vi "PicoScope6000aGetStreamingValues.vi"(0 "handle in":i16=16384, 1 "Polling time ms":u32=10, 2 "Buffer and Transfer Settings":T5={"startIndex"=0, "Samples"=1000000, "Down Sample Ratio"=1, "Down-Sample Mode"=2147483648} {"Down-Sample Mode" items=["RAW none"=2147483648, "None"=0, "Aggregate"=1, "Decimate"=2, "Average"=4]; "Down Sample Ratio" step=1; "Samples" format="%_6p"}, 3 "enabled array":i16[](array[numeric])=[1, 1, 0, 0, 0, 0, 0, 0, 0, 0], 5 "Device Info":T2, 7 "Data Pointers In":T3, 9 "No of Buffers":i32=1, 11 "error in (no error)":errorcluster, 13 "LoopFlag":bool) -> (4 "handle out":i16=16384, 8 "Data Pointers Out":T3, 14 "tPicoStreamingDataTriggerInfo":T1(array[cluster]), 15 "error out":errorcluster)   [LabVIEW 2010]
doc: "Call ps6000aGetValues to fill all buffers"
uses:
  ps6000a.dll
  shared/PicoBuffers.ctl
  shared/Buffer and Transfer Settings.ctl
panel:
  out "handle RunStreaming":i16
  out "error out RunStreaming":errorcluster
  out "No of channels":u64=2
  in  "tPicoStreamingDataInfo":T4={"Channel"=0, "Down-Sample Mode"=2147483648, "PICO_DATA_TYPE"=enum."PICO_INT16_T", "Samples"=0, "bufferIndex"=0, "startIndex"=0, "overflow"=0} {"overflow" step=1 format="%010b"; "Down-Sample Mode" items=["None"=2147483648, "Aggregate"=1, "Decimate"=2, "Average"=4]; "Channel" items=["Channel A"=0, "Channel B"=1, "Channel C"=2, "Channel D"=3, "Channel E"=4, "Channel F"=5, "Channel G"=6, "Channel H"=7, "Port 0"=128, "Port 1"=129, "Trigger AUX"=1001]; "startIndex" step=1}
  in  "SetDataBuffer0 flag":bool
  in  "Streaming Acquisition Settings":T6={"preTriggerSamples"=0, "postTriggerSamples"=1000000, "Requested sampleInterval"=1.0, "sampleIntervalTimeUnits"=3} {"sampleIntervalTimeUnits" items=["femtoseconds", "picoseconds", "nanoseconds", "microseconds", "millseconds", "seconds"]; "postTriggerSamples" format="%_6p"; "preTriggerSamples" format="%_6p"}
  # "Samples can be equal to or less\nTotal Pre and Post Trigger Samples"
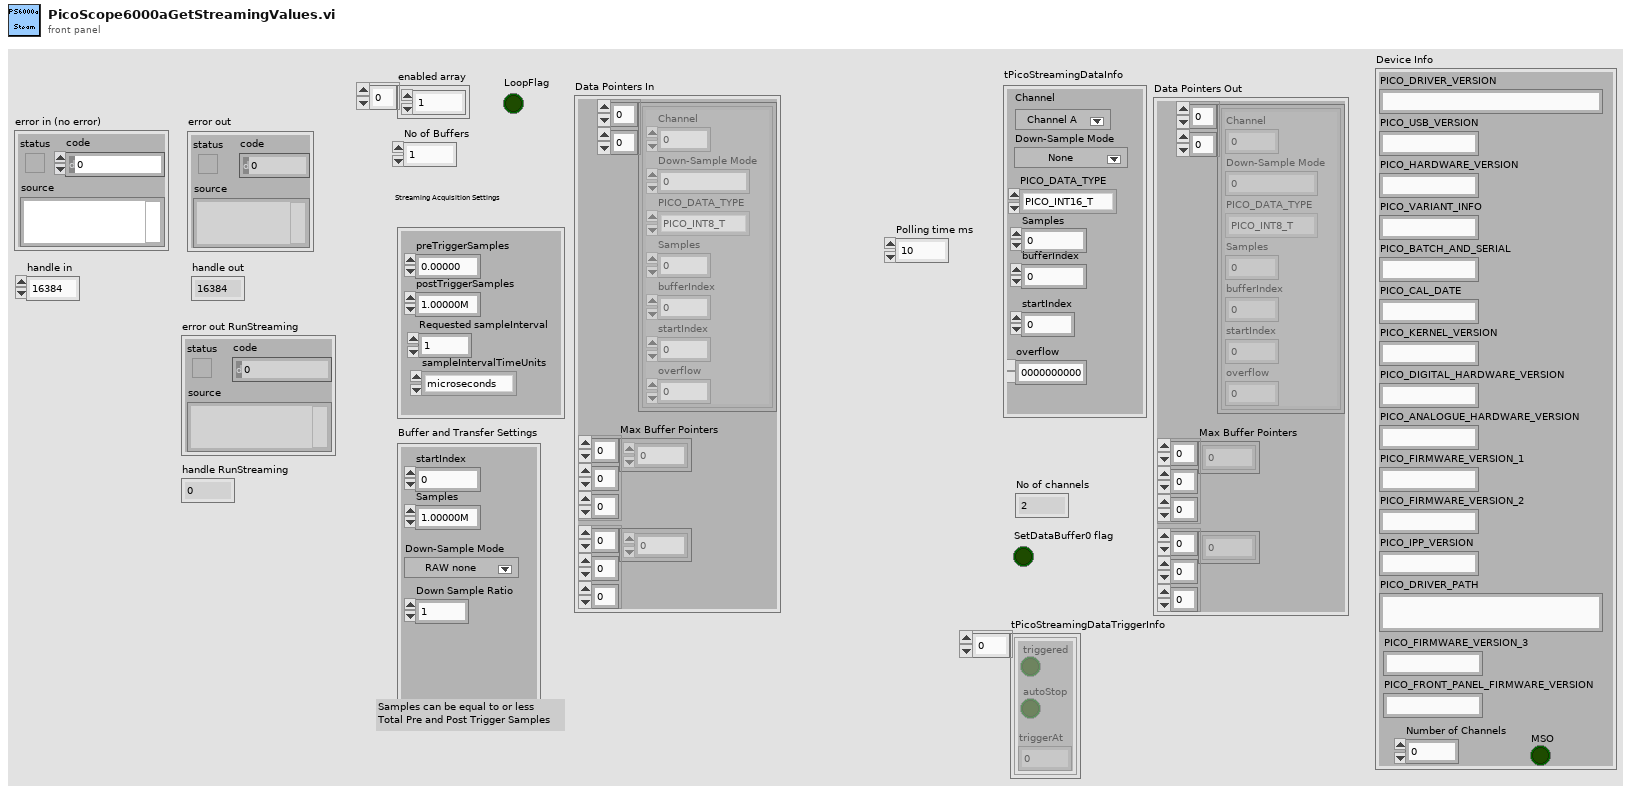
[diagram p1: front panel]
types:
  T1 = cluster{"triggerAt":u64, "triggered":bool, "autoStop":bool}[]
  T2 = cluster{"PICO_DRIVER_VERSION":string, "PICO_USB_VERSION":string, "PICO_HARDWARE_VERSION":string, "PICO_VARIANT_INFO":string, "PICO_BATCH_AND_SERIAL":string, "PICO_CAL_DATE":string, "PICO_KERNEL_VERSION":string, "PICO_DIGITAL_HARDWARE_VERSION":string, "PICO_ANALOGUE_HARDWARE_VERSION":string, "PICO_FIRMWARE_VERSION_1":string, "PICO_FIRMWARE_VERSION_2":string, "PICO_IPP_VERSION":string, "PICO_DRIVER_PATH":string, "PICO_FIRMWARE_VERSION_3":string, "PICO_FRONT_PANEL_FIRMWARE_VERSION":string, "Number of Channels":i16, "MSO":bool}
  T3 = typedef "PicoBuffers.ctl" = cluster{"Max Buffer Pointers":u64[][][], "Min Buffer Pointers":u64[][][], "StreamingDataInfo":cluster{"Channel":u32, "Down-Sample Mode":u32, "PICO_DATA_TYPE":enum32{"PICO_INT8_T", "PICO_INT16_T", "PICO_INT32_T", "PICO_UINT32_T", "PICO_INT64_T", ""}, "Samples":i32, "bufferIndex":u64, "startIndex":i32, "overflow":i16}[][]}
  T4 = cluster{"Channel":u32, "Down-Sample Mode":u32, "PICO_DATA_TYPE":enum32{"PICO_INT8_T", "PICO_INT16_T", "PICO_INT32_T", "PICO_UINT32_T", "PICO_INT64_T", ""}, "Samples":i32, "bufferIndex":u64, "startIndex":i32, "overflow":i16}
  T5 = typedef "Buffer and Transfer Settings.ctl" = cluster{"startIndex":u64, "Samples":u64, "Down Sample Ratio":u64, "Down-Sample Mode":u32}
  T6 = cluster{"preTriggerSamples":u64, "postTriggerSamples":u64, "Requested sampleInterval":dbl, "sampleIntervalTimeUnits":u32}
  T7 = enum32{"PICO_INT8_T", "PICO_INT16_T", "PICO_INT32_T", "PICO_UINT32_T", "PICO_INT64_T", ""}
  T8 = cluster{"triggerAt_":u64, "triggered_":i16, "autoStop_":i16}
  T9 = cluster{"Channel":u32, "Down-Sample Mode":u32, "PICO_DATA_TYPE":enum32{"PICO_INT8_T", "PICO_INT16_T", "PICO_INT32_T", "PICO_UINT32_T", "PICO_INT64_T", ""}, "Samples":i32, "bufferIndex":u64, "startIndex":i32, "overflow":i16}[]
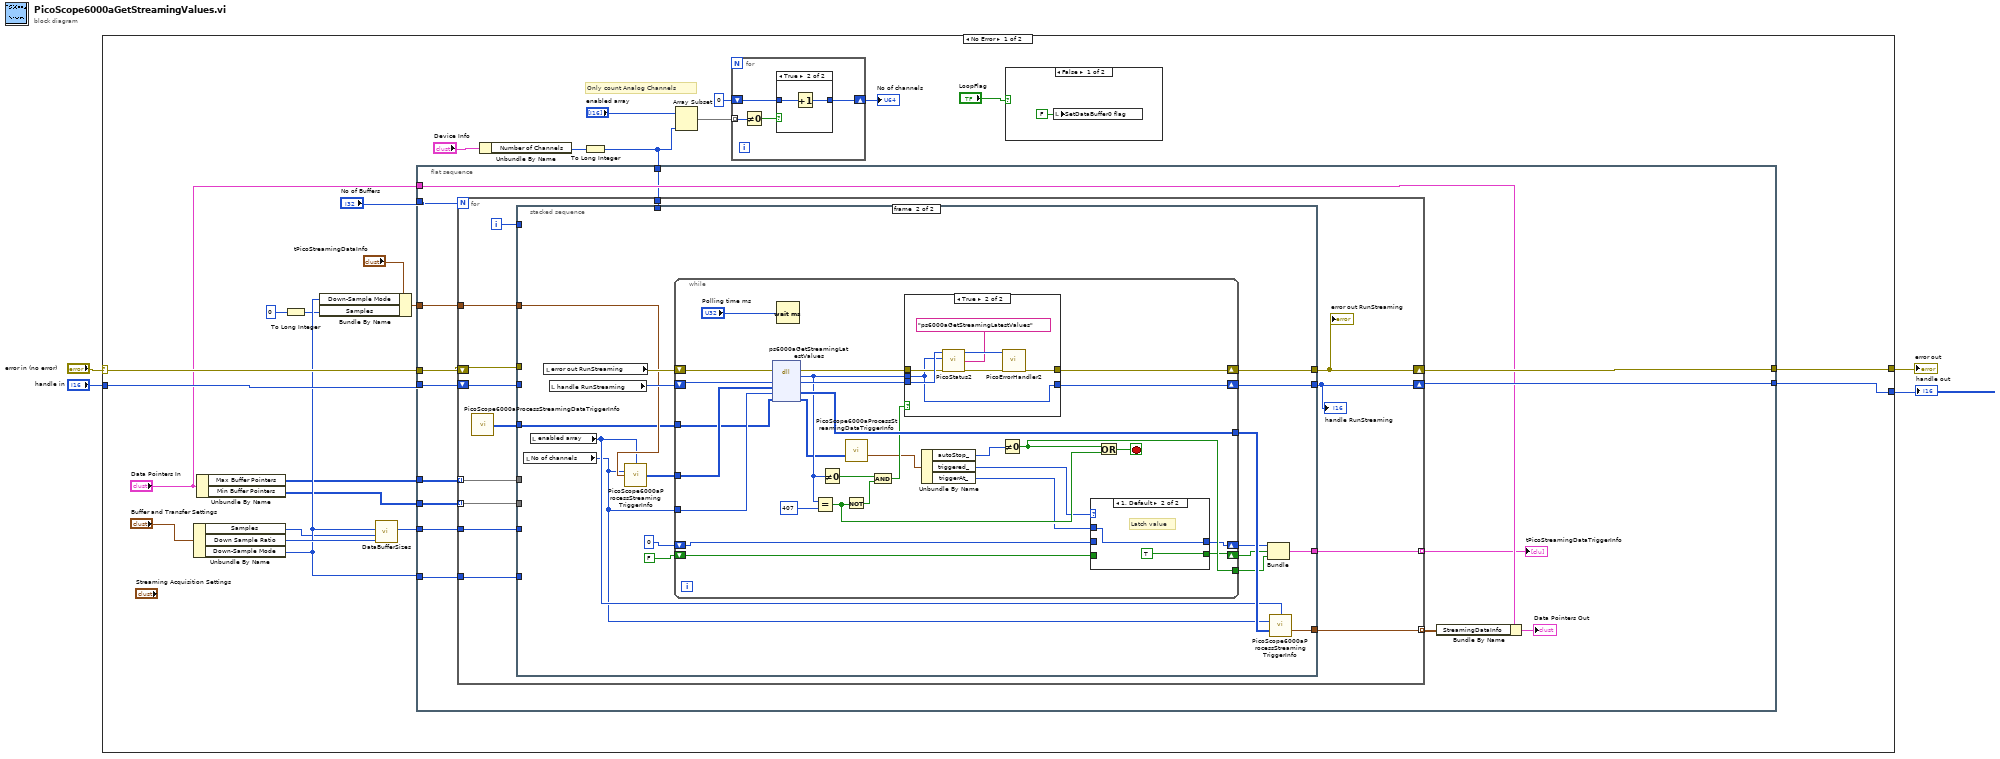
[diagram p0: block diagram]
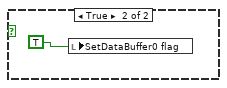
[diagram p2: hidden frame]
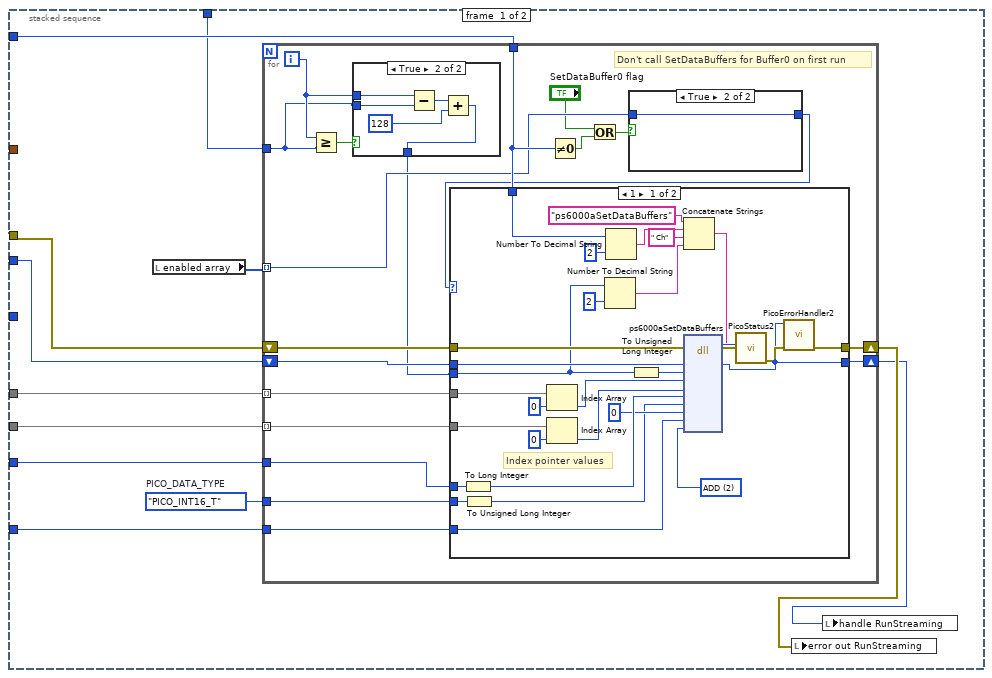
[diagram p4: hidden frame]
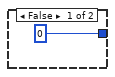
[diagram p6: hidden frame]
diagram:
  n1 = case shown="No Error" "error in (no error)" {
    selector: "error in (no error)" -> [w26 w196]
    tunnel: "handle in" -> [w25 w197]
    tunnel: [w29 w197] -> w2
    tunnel: [w27 w196] -> w1
    frame No Error {
      # "Only count Analog Channels"
      n2 = Unbundle By Name("Buffer and Transfer Settings") -> ("Samples"=w17:u64, "Down Sample Ratio"=w24:u64, "Down-Sample Mode"=w19:u32)
      n3 = Unbundle By Name("Data Pointers In") -> ("Max Buffer Pointers"=w14:u64[][][], "Min Buffer Pointers"=w13:u64[][][])
      n4 = To Long Integer(number=0) -> (32bit integer=w18:i32)
      n5 = Bundle By Name(cluster="tPicoStreamingDataInfo", "Down-Sample Mode"=w19, "Samples"=w18) -> (w20:T4)
      n6 = call "DataBufferSizes.vi"("Down Sample Ratio"=w24, "Number of Samples"=w17, "Down-Sample Mode"=w19) -> ("Max Buffer Size"=w22:i32)  [unwired: 7 in, 1 out]
      n7 = flat-sequence {
        tunnel: w26 -> [w50]
        tunnel: w25 -> [w47]
        tunnel: "No of Buffers" -> [w53]
        tunnel: w14 -> [w45]
        tunnel: w19 -> [w52]
        tunnel: w22 -> [w51]
        tunnel: w20 -> [w48]
        tunnel: w13 -> [w44]
        tunnel: [w46] -> w29
        tunnel: [w49] -> w27
        tunnel: "Data Pointers In" -> [w43]
        tunnel: w8 -> [w40]
        frame #0 {
          n8 = for {
            N: w53 -> [_]
            tunnel: w45 -> [w59] mode=indexing
            tunnel: w52 -> [w67]
            tunnel: w51 -> [w66]
            shift-right: [w64] -> w49
            shift-left: w50 -> [w65]
            tunnel: w48 -> [w63]
            shift-right: [w62] -> w46
            shift-left: w47 -> [w61]
            tunnel: w44 -> [w58] mode=indexing
            tunnel: [w57] -> w41 mode=indexing
            tunnel: w40 -> [w55]
            tunnel: [w54] -> w39 mode=indexing
            i -> [w60]
            n9 = call "PicoScope6000aProcessStreamingDataTriggerInfo.vi"() -> ("C Array for Struture Data Out"=w56:u16[][])  [unwired: 13 in, 2 out]
            n10 = stacked-sequence {
              tunnel: [_ w153] -> w62
              tunnel: w65 -> [w75 _]
              tunnel: w61 -> [w79 _]
              tunnel: w59 -> [w71 _]
              tunnel: w67 -> [w78 _]
              tunnel: w66 -> [w77 _]
              tunnel: w60 -> [w72 _]
              tunnel: [_ w152] -> w64
              tunnel: w63 -> [_ w151]
              tunnel: w58 -> [w69 _]
              tunnel: [_ w149] -> w57
              tunnel: w56 -> [_ w145]
              tunnel: w55 -> [w68 _]
              tunnel: [_ w144] -> w54
              frame #0 {
                w70 = T7."PICO_INT16_T"  # PICO_DATA_TYPE
                n11 = local read "enabled array"() -> (w76:i16[])
                n12 = for {
                  tunnel: w78 -> [w98]
                  tunnel: w70 -> [w97]
                  tunnel: w77 -> [w94]
                  tunnel: w76 -> [w90] mode=indexing
                  tunnel: w72 -> [w93]
                  shift-right: [w92] -> w74
                  shift-left: w75 -> [w96]
                  shift-right: [w91] -> w73
                  shift-left: w79 -> [w95]
                  tunnel: w71 -> [w85] mode=indexing
                  tunnel: w69 -> [w84] mode=indexing
                  tunnel: w68 -> [w80]
                  i -> [w81]
                  # "Don't call SetDataBuffers for Buffer0 on first run"
                  n13 = Greater Or Equal?(x=w81, y=w80) -> (x >= y?=w83:bool)
                  n14 = case shown="True" w83 {
                    tunnel: [w99 w103] -> w82
                    tunnel: w80 -> [_ w102]
                    tunnel: w81 -> [w99 w101]
                    frame False {
                    }
                    frame True {
                      n15 = Subtract(x=w101, y=w102) -> (x-y=w100:i32)
                      n16 = Add(x=w100, y=128) -> (x+y=w103:i32)
                    }
                  }
                  n17 = Not Equal To 0?(x=w93) -> (x != 0?=w88:bool)
                  n18 = Or(x="SetDataBuffer0 flag", y=w88) -> (x .or. y?=w86:bool)
                  n19 = case shown="True" w86 {
                    tunnel: [i16 0 ("element") w106] -> w89
                    tunnel: w90 -> [_ w106]
                    frame False {
                    }
                    frame True {
                    }
                  }
                  n20 = case shown="1" w89 {
                    tunnel: w82 -> [w115 _]
                    tunnel: w96 -> [w136 w138]
                    tunnel: w95 -> [w133 w137]
                    tunnel: w98 -> [w131 _]
                    tunnel: w97 -> [w109 _]
                    tunnel: w94 -> [w130 _]
                    tunnel: w85 -> [w114 _]
                    tunnel: [w128 w138] -> w92
                    tunnel: w93 -> [w123 _]
                    tunnel: [w119 w137] -> w91
                    tunnel: w84 -> [w107 _]
                    frame 1 {
                      w113 = u32 2 items=["NONE"=0, "CLEAR_ALL"=1, "ADD"=2, "CLEAR_THIS_DATA_BUFFER"=4096, "CLEAR_WAVEFORM_DATA_BUFFERS"=8192, "CLEAR_WAVEFORM_READ_DATA_BUFFERS"=16384] ("PicoAction 3")
                      # "Index pointer values"
                      n21 = To Long Integer(number=w130) -> (32bit integer=w129:i32)
                      n22 = To Unsigned Long Integer(number=w109) -> (unsigned 32bit integer=w108:u32)
                      n23 = Index Array(array=w114, index=0) -> (element=w117:u64)
                      n24 = Index Array(array=w107, index=0) -> (element=w110:u64)
                      n25 = Number To Decimal String(number=w115, width (-)=i16 2) -> (decimal integer string=w120:string)
                      n26 = Number To Decimal String(number=w123, width (-)=i16 2) -> (decimal integer string=w125:string)
                      n27 = To Unsigned Long Integer(number=w115) -> (unsigned 32bit integer=w116:u32)
                      n28 = Concatenate Strings("ps6000aSetDataBuffers" ("source"), w125, " Ch" ("string"), w120) -> (w126:string)
                      n29 = dll-call lib="ps6000a.dll" fn="ps6000aSetDataBuffers" ("ps3000.dll:_ps3000_open_unit@0")(error in=w136, "handle"=w133, "channel"=w116, "bufferMax"=w117, "bufferMin"=w110, "nSamples"=w129, "dataType"=w108, "waveform"=u64 0, "downSampleRatioMode"=w131, "action"=w113) -> (error out=w135:errorcluster, "PICO_STATUS"=w134:u32, "handle"=w119:i16)  [unwired: 10 in, 1 out]
                      n30 = call "PicoStatus2.vi"("PICO source"=w126, "Error in"=w135, "PICO STATUS"=w134) -> ("error out"=w132:errorcluster)  [unwired: 5 in, 1 out]
                      n31 = call "PicoErrorHandler2.vi"("error in (no error)"=w132, "handle In"=w119) -> ("error out"=w128:errorcluster)  [unwired: 9 in]
                    }
                    frame 0, Default {
                    }
                  }
                }
                n32 = local write "error out RunStreaming"(w74) -> ()
                n33 = local write "handle RunStreaming"(w73) -> ()
              }
              frame #1 {
                n34 = local read "No of channels"() -> (w146:u64)
                n35 = local read "enabled array"() -> (w147:i16[])
                n36 = local read "error out RunStreaming"() -> (w155:errorcluster)
                n37 = local read "handle RunStreaming"() -> (w154:i16)
                n38 = call "PicoScope6000aProcessStreamingTriggerInfo.vi"("enabled array"=w147, "No of C Strutures"=w146, "C Struture define"=w151) -> ("C Array for Struture Data Out"=w150:u16[][])  [unwired: 10 in, 2 out]
                n39 = while {
                  shift-right: [w181] -> w152
                  shift-left: w155 -> [w183]
                  shift-right: [w156] -> w153
                  shift-left: w154 -> [w182]
                  tunnel: w146 -> [w178]
                  tunnel: w150 -> [w177]
                  tunnel: [w176] -> w148
                  tunnel: w145 -> [w165]
                  tunnel: [w161] -> w143
                  shift-right: [w158] -> w139
                  shift-left: u64 0 ("triggerAt_") -> [w159]
                  shift-right: [w157] -> w140
                  shift-left: FALSE ("x = y?") -> [w160]
                  stop <- w166 stop-if-true
                  n40 = dll-call lib="ps6000a.dll" fn="ps6000aGetStreamingLatestValues" ("ps3000.dll:_ps3000_open_unit@0")(error in=w183, "handle"=w182, "streamingDataInfo"=w177, "nStreamingDataInfos"=w178, "triggerInfo"=w165) -> (error out=w180:errorcluster, "PICO_STATUS"=w174:u32, "handle"=w179:i16, "streamingDataInfo"=w176:u16[][], "triggerInfo"=w170:u16[][])  [unwired: 3 in, 1 out]
                  n41 = Wait (ms)(milliseconds to wait="Polling time ms") -> ()  [unwired: 1 out]
                  n42 = Equal?(x=w174, y=u32 407) -> (x = y?=w167:bool)
                  n43 = Not Equal To 0?(x=w174) -> (x != 0?=w172:bool)
                  n44 = Not(x=w167) -> (.not. x?=w171:bool)
                  n45 = call "PicoScope6000aProcessStreamingDataTriggerInfo.vi"("C Array for Struture Data In"=w170) -> ("tPicoStreamingDataTriggerInfo"=w169:T8)  [unwired: 12 in, 2 out]
                  n46 = And(x=w172, y=w171) -> (x .and. y?=w173:bool)
                  n47 = case shown="True" w173 {
                    tunnel: w179 -> [w188 w195]
                    tunnel: [w189 w194] -> w181
                    tunnel: w174 -> [_ w190]
                    tunnel: w180 -> [w189 w193]
                    tunnel: [w188 w190] -> w156
                    frame False {
                    }
                    frame True {
                      n48 = call "PicoStatus2.vi"("PICO source"="ps6000aGetStreamingLatestValues" ("source"), "Error in"=w193, "PICO STATUS"=w190) -> ("error out"=w191:errorcluster)  [unwired: 5 in, 1 out]
                      n49 = call "PicoErrorHandler2.vi"("error in (no error)"=w191, "handle In"=w195) -> ("error out"=w194:errorcluster)  [unwired: 9 in]
                    }
                  }
                  n50 = Unbundle By Name(w169) -> ("autoStop_"=w168:i16, "triggered_"=w163:i16, "triggerAt_"=w162:u64)
                  n51 = Not Equal To 0?(x=w168) -> (x != 0?=w161:bool)
                  n52 = case shown="1, Default" w163 {
                    tunnel: w159 -> [w184 _]
                    tunnel: [w184 w186] -> w158
                    tunnel: w160 -> [w185 _]
                    tunnel: [w185 TRUE ("x = y?")] -> w157
                    tunnel: w162 -> [_ w186]
                    frame 0 {
                    }
                    frame 1, Default {
                      # "Latch value"
                    }
                  }
                  n53 = Or(x=w161, y=w167) -> (x .or. y?=w166:bool)
                }
                n54 = Bundle("triggerAt_"=w139, "x = y?"=w140, w143) -> (w144:cluster{"triggerAt_":u64, "x = y?":bool, bool})  [unwired: 1 in]
                n55 = call "PicoScope6000aProcessStreamingTriggerInfo.vi"("enabled array"=w147, "No of C Strutures"=w146, "C Array for Struture Data In"=w148) -> ("Array of Clusters"=w149:T9)  [unwired: 10 in, 2 out]
              }
            }
            "error out RunStreaming" <- w64
            "handle RunStreaming" <- w62
          }
          "tPicoStreamingDataTriggerInfo" <- w39
          n56 = Bundle By Name(cluster=w43, "StreamingDataInfo"=w41) -> (→"Data Pointers Out":T3)
        }
      }
      n57 = Unbundle By Name("Device Info") -> ("Number of Channels"=w10:i16)
      n58 = To Long Integer(number=w10) -> (32bit integer=w8:i32)
      n59 = Array Subset(array="enabled array", length=w8) -> (w6:i16[])  [unwired: 1 in]
      n60 = for {
        shift-right: [w35] -> w5
        shift-left: u64 0 -> [w34]
        tunnel: w6 -> [w33] mode=indexing
        n61 = Not Equal To 0?(x=w33) -> (x != 0?=w32:bool)
        n62 = case shown="True" w32 {
          tunnel: [w36 w38] -> w35
          tunnel: w34 -> [w36 w37]
          frame False {
          }
          frame True {
            n63 = Increment(x=w37) -> (x+1=w38:u64)
          }
        }
      }
      "No of channels" <- w5
      n64 = case shown="False" "LoopFlag" {
        frame False {
          n65 = local write "SetDataBuffer0 flag"(FALSE ("SetDataBuffer0 flag")) -> ()
        }
        frame True {
          n66 = local write "SetDataBuffer0 flag"(TRUE ("SetDataBuffer0 flag")) -> ()
        }
      }
    }
    frame Error {
    }
  }
  "handle out" <- w2
  "error out" <- w1
